vi "End.vi"(8 "error in (no error)":errorcluster, 11 "AG in":refnum<class "AG.lvclass">) -> (0 "error out":errorcluster, 3 "AG out":refnum<class "AG.lvclass">)   [LabVIEW 2018]
uses:
  AG.lvclass
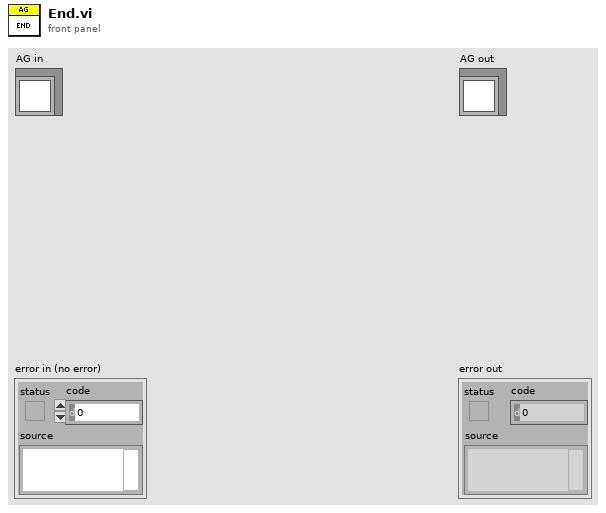
[diagram p1: front panel]
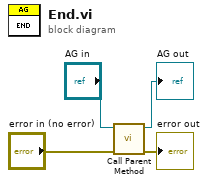
[diagram p0: block diagram]
diagram:
  n1 = call-parent "Call Parent Method"("error in (no error)"="error in (no error)", "Server in"="AG in") -> ("error out"=→"error out":errorcluster, "Server out"=→"AG out":refnum<class "AG.lvclass">)  [unwired: 8 in]
